vi "OnDemandWaveformDataBroadcast_Send.vi"(8 "error in (no error)":errorcluster, 10 "On Demand Waveform":T1, 11 "Qbus":refnum<class "Qbus.lvclass">) -> (0 "error out":errorcluster, 3 "Qbus out":refnum<class "Qbus.lvclass">)   [LabVIEW 2017, in "EmsaAcquisition.lvlib"]
uses:
  <vilib>/addons/InsightCM/Devices/Shared/Emsa/EmsaAcquisition/EmsaAcquisition.lvlib
  <vilib>/addons/Qbus/Qbus.lvclass
  <vilib>/addons/InsightCM/Devices/Shared/Emsa/EmsaAcquisition/controls/OnDemandWaveformData.ctl
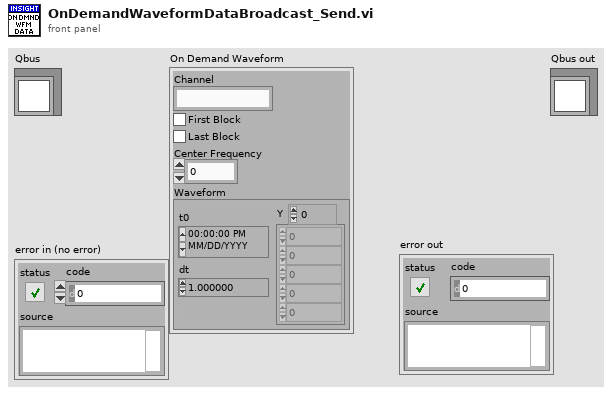
[diagram p1: front panel]
types:
  T1 = typedef "EmsaAcquisition.lvlib/OnDemandWaveformData.ctl" = cluster{"Channel":string, "First Block":bool, "Last Block":bool, "Center Frequency":dbl, "Waveform":waveform(dbl)}
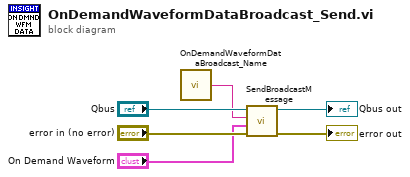
[diagram p0: block diagram]
diagram:
  n1 = call <vilib>:"OnDemandWaveformDataBroadcast_Name.vi"() -> ("message name"=w4:string)  [unwired: 5 in]
  n2 = call <vilib>:"SendBroadcastMessage.vi"("error in (no error)"="error in (no error)", "message value"="On Demand Waveform", "message name"=w4, "Qbus in"="Qbus") -> ("error in (no error)"=→"error out":errorcluster, "Qbus out"=→"Qbus out":refnum<class "Qbus.lvclass">)  [unwired: 6 in]
